vi "Control_Panel_정리.vi"() -> ()   [LabVIEW 2014]
panel:
  in  "Dump":dbl[](array[numeric])=[32.0, 29.0, 32.0, 32.0, 32.0, 32.0, 32.0, 32.0, 32.0, 32.0, 29.0, 32.0, 32.0, 32.0, 32.0, 32.0, 32.0, 32.0, 32.0, 32.0, 32.0, 32.0, 32.0, 32.0, 32.0, 32.0, 32.0, 32.0, 32.0, 32.0, 32.0, 32.0, 32.0, 32.0, 32.0, 32.0, 32.0, 32.0, 32.0, 32.0, 32.0, 32.0, 32.0, 33.0, 32.0, 32.0, 32.0, 32.0, 32.0, 32.0, 32.0, 32.0, 32.0, 32.0, 32.0, 32.0, 32.0, 32.0, 32.0, 33.0, 32.0, 32.0, 32.0, 32.0, 33.0, 33.0, 33.0, 32.0, 33.0, 32.0, 32.0, 32.0, 33.0, 33.0, 32.0, 33.0, 32.0, 32.0, 33.0, 32.0, 32.0, 33.0, 33.0, 33.0, 33.0, 33.0, 32.0, 32.0, 33.0, 33.0, 32.0, 33.0, 33.0, 32.0, 32.0, 33.0, 32.0, 32.0, 32.0, 33.0, 32.0, 32.0, 32.0, 33.0, 32.0, 32.0, 32.0, 33.0, 33.0, 32.0, 32.0, 33.0, 32.0, 33.0, 33.0, 33.0, 32.0, 32.0, 32.0, 33.0, 33.0, 32.0, 33.0, 32.0, 32.0, 33.0, 33.0, 33.0, 32.0, 33.0, 33.0, 32.0, 33.0, 33.0, 33.0, 33.0, 32.0, 32.0, 32.0, 32.0, 33.0, 32.0, 32.0, 33.0, 33.0, 32.0, 33.0, 32.0, 32.0, 32.0, 32.0, 33.0, 33.0, 32.0, 32.0, 32.0, 32.0, 32.0, 33.0, 33.0, 33.0, 32.0, 33.0, 32.0, 32.0, 32.0, 32.0, 32.0, 33.0, 33.0, 33.0, 33.0, 32.0, 33.0, 33.0, 33.0, 32.0, 33.0, 33.0, 33.0, 32.0, 32.0, 33.0, 33.0, 32.0, 32.0, 32.0, 33.0, 33.0, 33.0, 32.0, 33.0, 33.0, 33.0, 32.0, 32.0, 32.0, 32.0, 32.0, 32.0, 32.0, 32.0, 33.0, 33.0, 33.0, 33.0, 32.0, 33.0, 33.0, 33.0, 32.0, 33.0, 32.0, 33.0, 33.0, 32.0, 32.0, 33.0, 33.0, 32.0, 32.0, 33.0, 32.0, 32.0, 33.0, 33.0, 32.0, 32.0, 32.0, 32.0, 33.0, 32.0, 33.0, 33.0, 33.0, 33.0, 33.0, 33.0, 33.0, 33.0, 55.0, 2047.0, 2047.0, 2047.0, 2047.0, -1099.0, -1046.0, -999.0, -906.0, 2047.0, 2047.0, 2047.0, 2047.0, -1015.0, -1862.0, -1784.0, -1713.0, 835.0, 2047.0, 2047.0, 2047.0, 2047.0, -2048.0, -2048.0, -2048.0, -1780.0, 2047.0, 2047.0, 2047.0, 2047.0, 661.0, -2048.0, -2048.0, -2048.0, 524.0, 2047.0, 2047.0, 2047.0, 2047.0, -2048.0, -2048.0, -2048.0, -2048.0, 2047.0, 2047.0, 2047.0, 2047.0, 777.0, -2048.0, -2048.0, -2048.0, -292.0, 2047.0, 2047.0, 2047.0, 2047.0, -2048.0, -2048.0, -2048.0, -2048.0, 2047.0, 2047.0, 2047.0, 2047.0, 2047.0, -2048.0, -2048.0, -2048.0, -426.0, 2047.0, 2047.0, 2047.0, 2047.0, -677.0, -2048.0, -2048.0, -2048.0, 2047.0, 2047.0, 2047.0, 2047.0, 2047.0, -2048.0, -2048.0, -2048.0, -2048.0, 2047.0, 2047.0, 2047.0, 2047.0, -1436.0, -2048.0, -2048.0, -2048.0, -28.0, 2047.0, 2047.0, 2047.0, 2047.0, 2047.0, 2047.0, 2047.0, 2047.0, -2048.0, -2048.0, -2048.0, -2048.0, -169.0, 2047.0, 2047.0, 2047.0, 2047.0, 2047.0, 2047.0, 1494.0, 2047.0, 2037.0, 1957.0, 1884.0, 1815.0, 1750.0, 1688.0, 1628.0, 1570.0, 1513.0, 1460.0, 1409.0, 1356.0, 1308.0, 1261.0, 1218.0, 1174.0, 1131.0, 1092.0, 1052.0, 1015.0, 979.0, 945.0, 912.0, 880.0, 848.0, 818.0, 789.0, 768.0, -390.0, -2048.0, -2048.0, -444.0, 1290.0, 1223.0, 1171.0, 1125.0, 1082.0, 1044.0, 1005.0, 970.0, 936.0, 903.0, 870.0, 839.0, 810.0, 785.0, -121.0, -2048.0, -2048.0, -198.0, 1379.0, 1316.0, 1265.0, 1217.0, 1172.0, 1129.0, 1090.0, 1049.0, 1012.0, 977.0, 940.0, 907.0, 875.0, 844.0, 816.0, 788.0, 759.0, 731.0, 707.0, 681.0, 658.0, 634.0, 613.0, 592.0, 570.0, 551.0, 532.0, 514.0, 497.0, 480.0, 464.0, 448.0, 432.0, 418.0, 403.0, 389.0, 375.0, 362.0, 352.0, 340.0, 328.0, 316.0, 307.0, 296.0, 288.0, 277.0, 267.0, 260.0, 250.0, 243.0, 234.0, 228.0, 219.0, 214.0, 208.0, 200.0, 194.0, 187.0, 183.0, 178.0, 171.0, 166.0, 162.0, 156.0, 152.0, 149.0, -373.0, -2048.0, -2048.0, -2048.0, -2048.0, 821.0, 1409.0, 231.0, -2048.0, -2048.0, -2048.0, -2048.0, -2048.0, -2048.0, -2048.0, -2048.0, -2048.0, -2048.0, -2048.0, -2048.0, -2048.0, -2048.0, -2048.0, -2048.0, -2048.0, -2046.0, -1974.0, -1901.0, -1831.0, -1765.0, -1701.0, -1637.0, -1576.0, -1516.0, -1430.0, 2047.0, 2047.0, 2047.0, 2047.0, 2047.0, 2047.0, 2047.0, 2047.0, 2047.0, 2047.0, 2047.0, 2047.0, 2047.0, 2047.0, 2047.0, 2047.0, 2047.0, 2047.0, 1980.0, 1911.0, 1844.0, 1779.0, 1715.0, 1654.0, 1594.0, 1539.0, 1482.0, 1430.0, 1380.0, 1333.0, 1285.0, 1202.0, 1200.0, 1152.0, 1110.0, 1073.0, 1037.0, 689.0, -2048.0, -2048.0, -2048.0, -615.0, 1075.0, 1202.0, 995.0, 778.0, 1016.0, 1267.0, 1201.0, 1147.0, 1105.0, 1064.0, 1026.0, 988.0, 953.0, 920.0, 888.0, 858.0, 832.0, 773.0, -55.0, -2048.0, -2048.0, -2048.0, -2048.0, -2048.0, -2048.0, -1974.0, 849.0, 2047.0, 2010.0, 1927.0, 1857.0, 1627.0, -770.0, -2048.0, -2048.0, -2048.0, -2048.0, -2048.0, -2048.0, -2048.0, -2048.0, -2048.0, -2048.0, -2048.0, -2048.0, -2048.0, -2048.0, -2048.0, -2041.0, -1223.0, 2047.0, 2047.0, 2047.0, 2047.0, 2047.0, 2047.0, 2047.0, 2047.0, 2047.0, 2047.0, 2047.0, 2047.0, 2047.0, 2047.0, 2047.0, 2005.0, 1933.0, 1865.0, 1799.0, 1736.0, 1674.0, 1613.0, 1557.0, 1500.0, 1448.0, 1397.0, 1347.0, 1299.0, 1252.0, 1207.0, 1164.0, 1123.0, 1082.0, 1045.0, 1008.0, 971.0, 937.0, 905.0, 872.0, 840.0, 810.0, 784.0, 755.0, 728.0, 704.0, 679.0, 653.0, 631.0, 610.0, 587.0, 568.0, 549.0, 530.0, 512.0, 493.0, 476.0, 460.0, 444.0, 428.0, 416.0, 402.0, 388.0, 374.0, 361.0, 348.0, 338.0, 326.0, 314.0, 306.0, 295.0, 285.0, 276.0, 267.0, 259.0, 249.0, 242.0, 233.0, 227.0, 219.0, 213.0, 205.0, 199.0, 194.0, 187.0, 181.0, 177.0, 170.0, 165.0, 161.0, 155.0, 151.0, 147.0, 141.0, 138.0, 134.0, 131.0, 128.0, 123.0, 120.0, 117.0, 114.0, 112.0, 106.0, 106.0, -1144.0, -2048.0, -2048.0, 696.0, 856.0, 817.0, 784.0, 755.0, 674.0, -2048.0, -2048.0, -2048.0, 1433.0, 1361.0, 1303.0, 1253.0, 1207.0, 1163.0, 1122.0, 1081.0, 1043.0, 1005.0, 970.0, 935.0, 902.0, 870.0, 840.0, 810.0, 780.0, 754.0, 728.0, 701.0, 677.0, 653.0, 631.0, 609.0, 587.0, 567.0, 548.0, 529.0, 512.0, 492.0, 475.0, 459.0, 443.0, 428.0, 413.0, 401.0, 387.0, 373.0, 360.0, 348.0, 337.0, 326.0, 314.0, 306.0, 296.0, 289.0, 278.0, 268.0, 260.0, 250.0, 242.0, 233.0, 227.0, 218.0, 213.0, 205.0, 199.0, 194.0, 186.0, 181.0, 177.0, 170.0, 165.0, 161.0, 155.0, 151.0, 147.0, 144.0, 138.0, 134.0, 131.0, 128.0, 122.0, 120.0, 117.0, 114.0, 112.0, 106.0, 104.0, 102.0, 100.0, 97.0, 93.0, 91.0, 89.0, 87.0, 86.0, 84.0, 82.0, 81.0, 77.0, 75.0, 74.0, 72.0, 71.0, 70.0, 69.0, 67.0, 67.0, 65.0, 64.0, 61.0, 59.0, 59.0, 58.0, 57.0, 56.0, 55.0, 54.0, 54.0, 53.0, 52.0, 52.0, 50.0, 51.0, 50.0, 49.0, 48.0, 48.0, 48.0, 45.0, 44.0, 44.0, 44.0, 44.0, 42.0, 42.0, 42.0, 41.0, 41.0, 41.0, 40.0, 40.0, 40.0, 39.0, 39.0, 39.0, 38.0, 38.0, 38.0, 38.0, 37.0, 37.0, 37.0, 37.0, 37.0, 37.0, 37.0, 36.0, 36.0, 36.0, 36.0, 35.0, 36.0, 35.0, 35.0, 35.0, 35.0, 35.0, 35.0, 34.0, 35.0, 34.0, 34.0, 34.0, 34.0, 34.0, 35.0, 35.0, 34.0, 36.0, 37.0, -1003.0, -2048.0, -2048.0, -2048.0, -2048.0, -2048.0, -2048.0, -2048.0, -2048.0, -2048.0, -2048.0, -2048.0, -840.0, 2047.0, 2047.0, 2047.0, 2047.0, 2047.0, 2047.0, 2047.0, 2000.0, 1929.0, 1861.0, 1795.0, 1732.0, 1670.0, 1610.0, 1554.0, 1497.0, 1444.0, 1393.0, 1344.0, 1296.0, 1250.0, 1204.0, 1161.0, 1121.0, 1080.0, 1042.0, 1004.0, 968.0, 934.0, 901.0, 869.0, 839.0, 809.0, 780.0, 754.0, 727.0, 701.0, 677.0, 652.0, 630.0, 609.0, 586.0, 566.0, 547.0, 529.0, 508.0, 492.0, 474.0, 458.0, 442.0, 428.0, 413.0, 401.0, 387.0, 373.0, 360.0, 348.0, 338.0, 326.0, 314.0, 306.0, 294.0, 284.0, 276.0, 266.0, 258.0, 249.0, 243.0, -715.0, -2048.0, -2048.0, -2048.0, -2048.0, 1416.0, 1349.0, 1296.0, 1249.0, 1131.0, -2048.0, -2048.0, 1429.0, 1341.0, 1282.0, 1228.0, 1181.0, 1140.0, 1097.0, 1059.0, 1020.0, 984.0, 950.0, 917.0, 884.0, 852.0, 823.0, 793.0, 765.0, 739.0, 712.0, 688.0, 663.0, 642.0, 617.0, 597.0, 577.0, 555.0, 536.0, 518.0, 500.0, 484.0, 467.0, 451.0, 435.0, 421.0, 406.0, 392.0, 378.0, 364.0, 354.0, 342.0, 330.0, 321.0, 309.0, 298.0, 289.0, 279.0, 272.0, 261.0, 252.0, 245.0, 236.0, 229.0, 221.0, 215.0, 209.0, 201.0, 197.0, 189.0, 184.0, 179.0, 172.0, 167.0, 163.0, 156.0, 152.0, 149.0, 145.0, 140.0, 136.0, 132.0, 129.0, 124.0, 120.0, 118.0, 115.0, 113.0, 108.0, 106.0, 103.0, 101.0, 99.0, 97.0, 93.0, 91.0, 88.0, 86.0, 85.0, 83.0, 81.0, 80.0, 76.0, 74.0, 73.0, 72.0, 70.0, 69.0, 68.0, 67.0, 66.0, 64.0, 64.0, 60.0, 59.0, 58.0, 57.0, 57.0, 56.0, 55.0, 54.0, 53.0, 53.0, 52.0, 51.0, 51.0, 50.0, 49.0, 49.0, 48.0, 48.0, 45.0, 45.0, 44.0, 44.0, 43.0, 42.0, 42.0, 42.0, 42.0, 41.0, 41.0, 40.0, 40.0, 39.0, 39.0, 39.0, 39.0, 38.0, 38.0, 38.0, 38.0, 38.0, 37.0, 37.0, 37.0, 37.0, 36.0, 36.0, 36.0, 36.0, 36.0, 36.0, 35.0, 35.0, 35.0, 35.0, 35.0, 34.0, 34.0, 35.0, 35.0, 35.0, 35.0, 34.0, 34.0, 34.0, 34.0, 34.0, 33.0, 34.0, 34.0, 33.0, 33.0, 34.0, 34.0, 33.0, 33.0, 33.0, 33.0, 33.0, 33.0, 33.0, 33.0, 33.0, 33.0, 33.0, 33.0, 33.0, 32.0, 32.0, 32.0, 32.0, 32.0, 32.0, 32.0, 32.0, 32.0, 32.0, 32.0, 32.0, 33.0, 33.0, 32.0, 32.0, 32.0, 32.0, 32.0, 32.0, 32.0, 32.0, 32.0, 32.0, 32.0, 29.0, 32.0, 32.0, 32.0, 32.0, 32.0, 32.0, 32.0]
  out "Connected":bool
  in  "Start":bool=TRUE
  out "Communication Stopped":bool
  out "Acquisition Mode":bool
  out "Device Control Enabled":bool
  in  "Value Achieving Status":string
  in  "Connection":string
  in  "Enable Blink Detection Err Code":string
  in  "Write DataLog Path":string
  in  "Set Data Log Path":string
  in  "Connection ID":string
  in  "선택된 기능":string="응급"
  in  "전체종료 여부":string
  in  "Brain":path
  in  "ERP_Parameters_of_NonTarget_prior":path=path "C:/Emotion_Research/MyungjooWon_Training_Test(LDA)/2014-06-19/ERP_Parameters_of_NonTarget_prior.txt"
  in  "ERP_Parameters_of_Target_prior":path=path "C:/Emotion_Research/MyungjooWon_Training_Test(LDA)/2014-06-19/ERP_Parameters_of_Target_prior.txt"
  in  "Maximum_Iteration":i64=100
  in  "in":path=path "C:/Emotion_Research/MyungjooWon_Training_Test(LDA)/2014-06-19/in_SWLDA.txt"
  in  "Fatigue_Threshold":path
  in  "EEG_Channel_Num":i32=1
  in  "rate":dbl=512.0 caption="Rate" format="%0.2f"
  in  "sample mode":i32(ring)=10123 items=["유한 샘플"=10178, "연속 샘플"=10123, "하드웨어 타이밍에 의한 단일 포인트"=12522]
  in  "input terminal configuration":i32(ring)=10078 items=["기본값"=-1, "RSE"=10083, "NRSE"=10078, "차동"=10106, "유사 차동"=12529]
  in  "physical channels":tag="cDAQ1Mod5/ai0:6"
  in  "Experimentation_num":i32=2
  in  "LDA_Matrix":path=path "C:/Emotion_Research/MyungjooWon_Training_Test(LDA)/2014-06-19/LDA_Matrix_Value_SWLDA.txt"
  in  "피험자 이름":string="MyungjooWon"
  in  "정지":bool
  in  "Frame Length":i32=20
  in  "Flash_Repeat":i32=20
  in  "Random_num":i32=6
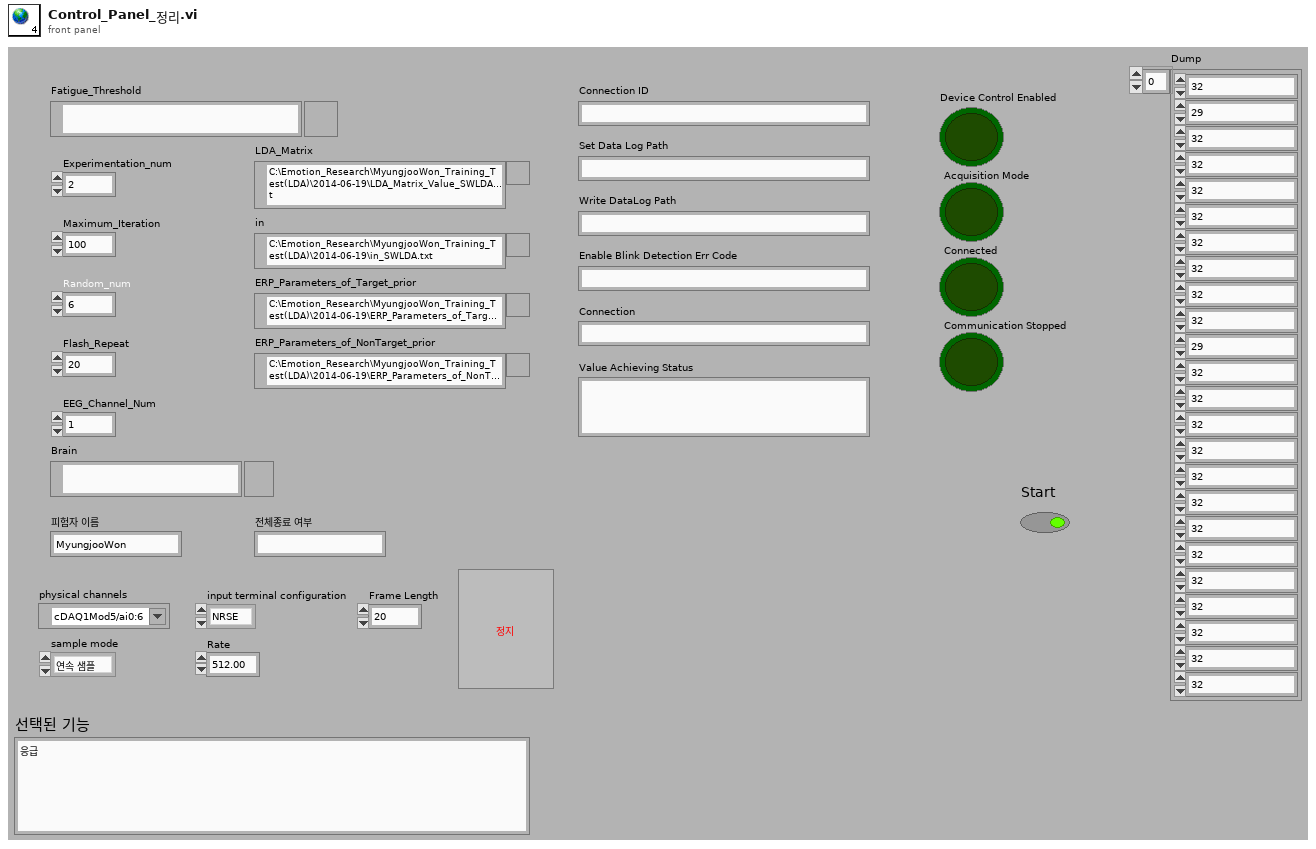
[diagram p1: front panel]
diagram:
